vi "1WIRE_MATCH_ROM.vi"(7 "1-Wire DIO Pin":refnum<k21>="ConnectorA/DIO15", 8 "error in (no error)":errorcluster, 10 "ROM Code":u64) -> (0 "error out":errorcluster)   [LabVIEW 2014]
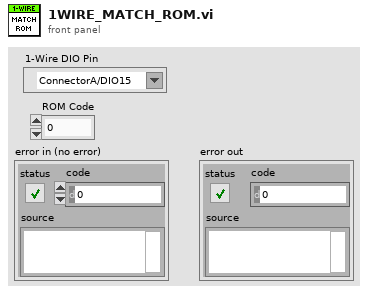
[diagram p1: front panel]
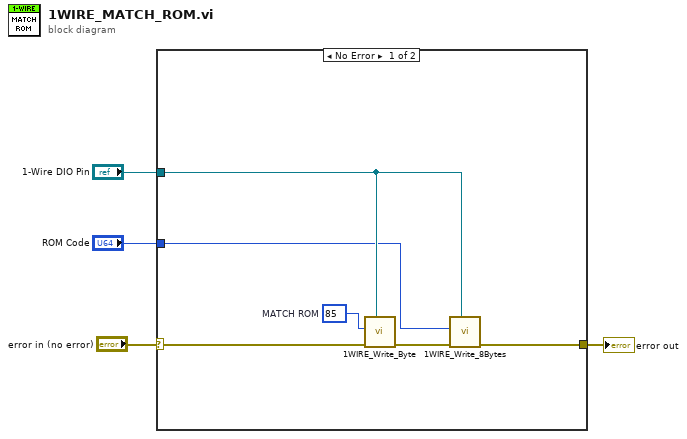
[diagram p0: block diagram]
diagram:
  n1 = case shown="No Error" "error in (no error)" {
    selector: "error in (no error)" -> [w9 w11]
    tunnel: [w7 w11] -> w4
    tunnel: "1-Wire DIO Pin" -> [w6 _]
    tunnel: "ROM Code" -> [w5 _]
    frame No Error {
      w10 = u8 85  # MATCH ROM
      n2 = call "1WIRE_Write_Byte.vi"("1-Wire DIO Pin"=w6, "error in"=w9, "Tx data"=w10) -> ("error out"=w8:errorcluster)  [unwired: 7 in, 1 out]
      n3 = call "1WIRE_Write_8Bytes.vi"("1-Wire DIO Pin"=w6, "error in"=w8, "Tx data"=w5) -> ("error out"=w7:errorcluster)  [unwired: 7 in, 1 out]
    }
    frame Error {
    }
  }
  "error out" <- w4
